vi "ConvertPatternTo64PinPGA.vi"(11 "Pattern":T10) -> (3 "64-Pin PGA":T1)   [LabVIEW 2012, in "Virtual-PGA.lvlib"]
uses:
  Virtual-PGA.lvlib
  Public/Controls/Pattern.ctl
  Public/Controls/Input.ctl
  Public/Controls/64PinPGAPattern.ctl
  Public/Controls/64PinPGAPads1-16.ctl
  Public/Controls/64PinPGAPad1-16.ctl
  Public/Controls/64PinPGAPads17-32.ctl
  Public/Controls/64PinPGAPad17-32.ctl
  Public/Controls/64PinPGAPads33-48.ctl
  Public/Controls/64PinPGAPad33-48.ctl
  Public/Controls/64PinPGAPads49-64.ctl
  Public/Controls/64PinPGAPad49-64.ctl
panel:
  # "Name:"
  # "Inputs:"
  # "Description:"
  # "Y4:"
  # "Y3:"
  # "Y2:"
  # "Y1:"
  # "49"
  # "50"
  # "51"
  # "52"
  # "53"
  # "54"
  # "55"
  # "56"
  # "57"
  # "58"
  # "59"
  # "60"
  # "61"
  # "62"
  # "63"
  # "64"
  # "1"
  # "2"
  # "3"
  # "4"
  # "5"
  # "6"
  # "7"
  # "8"
  # "9"
  # "10"
  # "11"
  # "12"
  # "13"
  # "14"
  # "15"
  # "16"
  # "32"
  # "31"
  # "30"
  # "29"
  # "28"
  # "27"
  # "26"
  # "25"
  # "24"
  # "23"
  # "22"
  # "21"
  # "20"
  # "19"
  # "18"
  # "17"
  # "48"
  # "47"
  # "46"
  # "45"
  # "44"
  # "43"
  # "42"
  # "41"
  # "40"
  # "39"
  # "38"
  # "37"
  # "36"
  # "35"
  # "34"
  # "33"
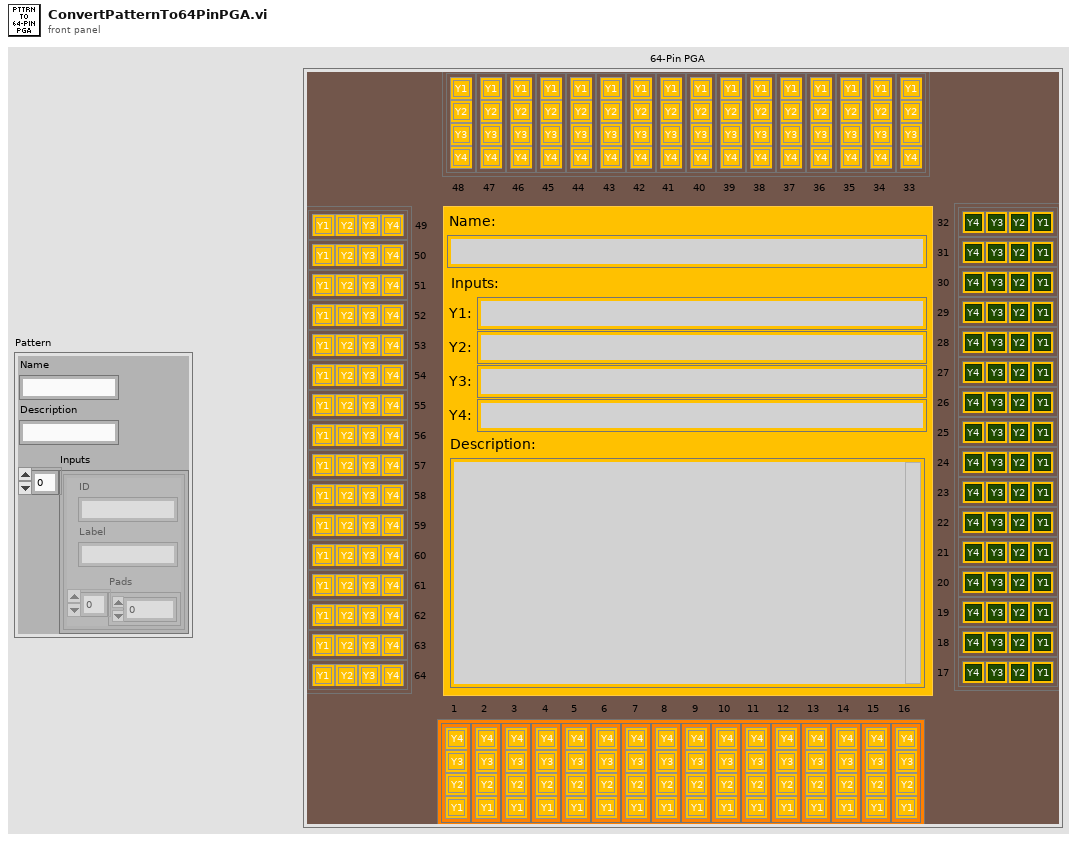
[diagram p1: front panel]
types:
  T1 = typedef "Virtual-PGA.lvlib/64PinPGAPattern.ctl" = cluster{"Name":string, "Description":string, "Y1 Label":string, "Y2 Label":string, "Y3 Label":string, "Y4 Label":string, "Pads 1-16":T2, "Pads 17-32":T4, "Pads 33-48":T6, "Pads 49-64":T8}
  T2 = typedef "Virtual-PGA.lvlib/64PinPGAPads1-16.ctl" = T3[]
  T3 = typedef "Virtual-PGA.lvlib/64PinPGAPad1-16.ctl" = cluster{"Y1":bool, "Y2":bool, "Y3":bool, "Y4":bool}
  T4 = typedef "Virtual-PGA.lvlib/64PinPGAPads17-32.ctl" = T5[]
  T5 = typedef "Virtual-PGA.lvlib/64PinPGAPad17-32.ctl" = cluster{"Y1":bool, "Y2":bool, "Y3":bool, "Y4":bool}
  T6 = typedef "Virtual-PGA.lvlib/64PinPGAPads33-48.ctl" = T7[]
  T7 = typedef "Virtual-PGA.lvlib/64PinPGAPad33-48.ctl" = cluster{"Y1":bool, "Y2":bool, "Y3":bool, "Y4":bool}
  T8 = typedef "Virtual-PGA.lvlib/64PinPGAPads49-64.ctl" = T9[]
  T9 = typedef "Virtual-PGA.lvlib/64PinPGAPad49-64.ctl" = cluster{"Y1":bool, "Y2":bool, "Y3":bool, "Y4":bool}
  T10 = typedef "Virtual-PGA.lvlib/Pattern.ctl" = cluster{"Name":string, "Description":string, "Inputs":T11[]}
  T11 = typedef "Virtual-PGA.lvlib/Input.ctl" = cluster{"ID":string, "Label":string, "Pads":u32[]}
  T12 = cluster{"Y1":bool, "Y2":bool, "Y3":bool, "Y4":bool}[]
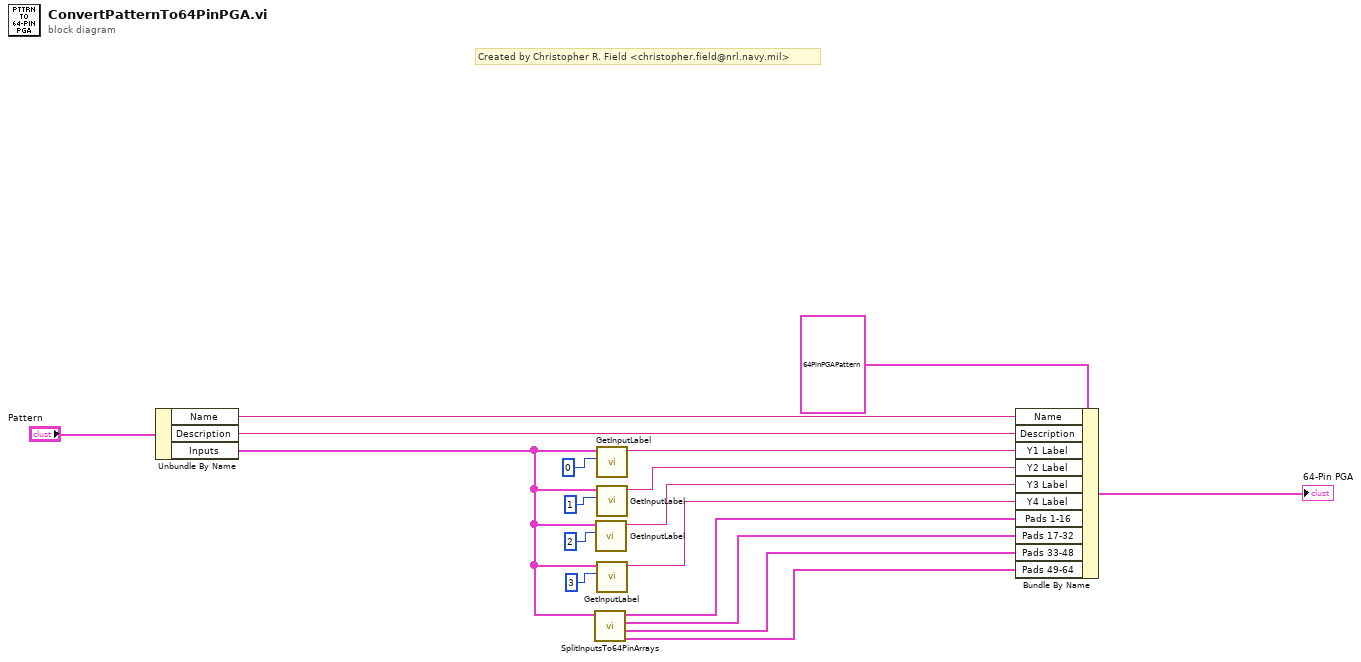
[diagram p0: block diagram]
diagram:
  # "Created by Christopher R. Field <christopher.field@nrl.navy.mil>"
  n1 = Unbundle By Name("Pattern") -> ("Name"=w15:string, "Description"=w14:string, "Inputs"=w5:T11[])
  n2 = call "SplitInputsTo64PinArrays.vi"("Inputs"=w5) -> ("Pads 49-64"=w1:T12, "Pads 33-48"=w2:T12, "Pads 17-32"=w3:T12, "Pads 1-16"=w4:T12)  [unwired: 7 in]
  n3 = call "GetInputLabel.vi"("Input Index"=2, "Inputs"=w5) -> ("Input Label"=w7:string)  [unwired: 9 in]
  n4 = call "GetInputLabel.vi"("Input Index"=0, "Inputs"=w5) -> ("Input Label"=w9:string)  [unwired: 9 in]
  n5 = call "GetInputLabel.vi"("Input Index"=1, "Inputs"=w5) -> ("Input Label"=w8:string)  [unwired: 9 in]
  n6 = call "GetInputLabel.vi"("Input Index"=3, "Inputs"=w5) -> ("Input Label"=w6:string)  [unwired: 9 in]
  n7 = Bundle By Name(cluster=T1 {"Name"="", "Description"="", "Y1 Label"="", "Y2 Label"="", "Y3 Label"="", "Y4 Label"="", "Pads 1-16"=[{"Y1"=FALSE, "Y2"=FALSE, "Y3"=FALSE, "Y4"=FALSE}, {"Y1"=FALSE, "Y2"=FALSE, "Y3"=FALSE, "Y4"=FALSE}, {"Y1"=FALSE, "Y2"=FALSE, "Y3"=FALSE, "Y4"=FALSE}, {"Y1"=FALSE, "Y2"=FALSE, "Y3"=FALSE, "Y4"=FALSE}, {"Y1"=FALSE, "Y2"=FALSE, "Y3"=FALSE, "Y4"=FALSE}, {"Y1"=FALSE, "Y2"=FALSE, "Y3"=FALSE, "Y4"=FALSE}, {"Y1"=FALSE, "Y2"=FALSE, "Y3"=FALSE, "Y4"=FALSE}, {"Y1"=FALSE, "Y2"=FALSE, "Y3"=FALSE, "Y4"=FALSE}, {"Y1"=FALSE, "Y2"=FALSE, "Y3"=FALSE, "Y4"=FALSE}, {"Y1"=FALSE, "Y2"=FALSE, "Y3"=FALSE, "Y4"=FALSE}, {"Y1"=FALSE, "Y2"=FALSE, "Y3"=FALSE, "Y4"=FALSE}, {"Y1"=FALSE, "Y2"=FALSE, "Y3"=FALSE, "Y4"=FALSE}, {"Y1"=FALSE, "Y2"=FALSE, "Y3"=FALSE, "Y4"=FALSE}, {"Y1"=FALSE, "Y2"=FALSE, "Y3"=FALSE, "Y4"=FALSE}, {"Y1"=FALSE, "Y2"=FALSE, "Y3"=FALSE, "Y4"=FALSE}, {"Y1"=FALSE, "Y2"=FALSE, "Y3"=FALSE, "Y4"=FALSE}], "Pads 17-32"=[{"Y1"=FALSE, "Y2"=FALSE, "Y3"=FALSE, "Y4"=FALSE}, {"Y1"=FALSE, "Y2"=FALSE, "Y3"=FALSE, "Y4"=FALSE}, {"Y1"=FALSE, "Y2"=FALSE, "Y3"=FALSE, "Y4"=FALSE}, {"Y1"=FALSE, "Y2"=FALSE, "Y3"=FALSE, "Y4"=FALSE}, {"Y1"=FALSE, "Y2"=FALSE, "Y3"=FALSE, "Y4"=FALSE}, {"Y1"=FALSE, "Y2"=FALSE, "Y3"=FALSE, "Y4"=FALSE}, {"Y1"=FALSE, "Y2"=FALSE, "Y3"=FALSE, "Y4"=FALSE}, {"Y1"=FALSE, "Y2"=FALSE, "Y3"=FALSE, "Y4"=FALSE}, {"Y1"=FALSE, "Y2"=FALSE, "Y3"=FALSE, "Y4"=FALSE}, {"Y1"=FALSE, "Y2"=FALSE, "Y3"=FALSE, "Y4"=FALSE}, {"Y1"=FALSE, "Y2"=FALSE, "Y3"=FALSE, "Y4"=FALSE}, {"Y1"=FALSE, "Y2"=FALSE, "Y3"=FALSE, "Y4"=FALSE}, {"Y1"=FALSE, "Y2"=FALSE, "Y3"=FALSE, "Y4"=FALSE}, {"Y1"=FALSE, "Y2"=FALSE, "Y3"=FALSE, "Y4"=FALSE}, {"Y1"=FALSE, "Y2"=FALSE, "Y3"=FALSE, "Y4"=FALSE}, {"Y1"=FALSE, "Y2"=FALSE, "Y3"=FALSE, "Y4"=FALSE}], "Pads 33-48"=[{"Y1"=FALSE, "Y2"=FALSE, "Y3"=FALSE, "Y4"=FALSE}, {"Y1"=FALSE, "Y2"=FALSE, "Y3"=FALSE, "Y4"=FALSE}, {"Y1"=FALSE, "Y2"=FALSE, "Y3"=FALSE, "Y4"=FALSE}, {"Y1"=FALSE, "Y2"=FALSE, "Y3"=FALSE, "Y4"=FALSE}, {"Y1"=FALSE, "Y2"=FALSE, "Y3"=FALSE, "Y4"=FALSE}, {"Y1"=FALSE, "Y2"=FALSE, "Y3"=FALSE, "Y4"=FALSE}, {"Y1"=FALSE, "Y2"=FALSE, "Y3"=FALSE, "Y4"=FALSE}, {"Y1"=FALSE, "Y2"=FALSE, "Y3"=FALSE, "Y4"=FALSE}, {"Y1"=FALSE, "Y2"=FALSE, "Y3"=FALSE, "Y4"=FALSE}, {"Y1"=FALSE, "Y2"=FALSE, "Y3"=FALSE, "Y4"=FALSE}, {"Y1"=FALSE, "Y2"=FALSE, "Y3"=FALSE, "Y4"=FALSE}, {"Y1"=FALSE, "Y2"=FALSE, "Y3"=FALSE, "Y4"=FALSE}, {"Y1"=FALSE, "Y2"=FALSE, "Y3"=FALSE, "Y4"=FALSE}, {"Y1"=FALSE, "Y2"=FALSE, "Y3"=FALSE, "Y4"=FALSE}, {"Y1"=FALSE, "Y2"=FALSE, "Y3"=FALSE, "Y4"=FALSE}, {"Y1"=FALSE, "Y2"=FALSE, "Y3"=FALSE, "Y4"=FALSE}], "Pads 49-64"=[{"Y1"=FALSE, "Y2"=FALSE, "Y3"=FALSE, "Y4"=FALSE}, {"Y1"=FALSE, "Y2"=FALSE, "Y3"=FALSE, "Y4"=FALSE}, {"Y1"=FALSE, "Y2"=FALSE, "Y3"=FALSE, "Y4"=FALSE}, {"Y1"=FALSE, "Y2"=FALSE, "Y3"=FALSE, "Y4"=FALSE}, {"Y1"=FALSE, "Y2"=FALSE, "Y3"=FALSE, "Y4"=FALSE}, {"Y1"=FALSE, "Y2"=FALSE, "Y3"=FALSE, "Y4"=FALSE}, {"Y1"=FALSE, "Y2"=FALSE, "Y3"=FALSE, "Y4"=FALSE}, {"Y1"=FALSE, "Y2"=FALSE, "Y3"=FALSE, "Y4"=FALSE}, {"Y1"=FALSE, "Y2"=FALSE, "Y3"=FALSE, "Y4"=FALSE}, {"Y1"=FALSE, "Y2"=FALSE, "Y3"=FALSE, "Y4"=FALSE}, {"Y1"=FALSE, "Y2"=FALSE, "Y3"=FALSE, "Y4"=FALSE}, {"Y1"=FALSE, "Y2"=FALSE, "Y3"=FALSE, "Y4"=FALSE}, {"Y1"=FALSE, "Y2"=FALSE, "Y3"=FALSE, "Y4"=FALSE}, {"Y1"=FALSE, "Y2"=FALSE, "Y3"=FALSE, "Y4"=FALSE}, {"Y1"=FALSE, "Y2"=FALSE, "Y3"=FALSE, "Y4"=FALSE}, {"Y1"=FALSE, "Y2"=FALSE, "Y3"=FALSE, "Y4"=FALSE}]} ("64-Pin PGA"), "Name"=w15, "Description"=w14, "Y1 Label"=w9, "Y2 Label"=w8, "Y3 Label"=w7, "Y4 Label"=w6, "Pads 1-16"=w4, "Pads 17-32"=w3, "Pads 33-48"=w2, "Pads 49-64"=w1) -> (→"64-Pin PGA":T1)
